vi "Define PDE Boundary Condition.vi"   [LabVIEW 2017, in "NI_PDE.lvlib"]
doc: "Defines the boundary condition of partial differential equations. You must manually select the polymorphic instance to use."
uses:
  <vilib>/gmath/NI_PDE.lvlib
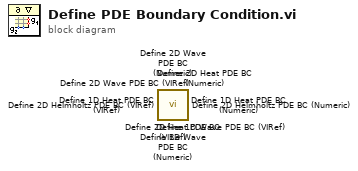
[diagram p0: block diagram]
diagram:
  n1 = call <vilib>:"Define 2D Heat PDE BC (VIRef).vi"() -> ()  [unwired: 14 in, 2 out]
  n2 = call <vilib>:"Define 2D Heat PDE BC (Numeric).vi"() -> ()  [unwired: 14 in, 2 out]
  n3 = call <vilib>:"Define 1D Heat PDE BC (VIRef).vi"() -> ()  [unwired: 14 in, 2 out]
  n4 = call <vilib>:"Define 1D Heat PDE BC (Numeric).vi"() -> ()  [unwired: 14 in, 2 out]
  n5 = call <vilib>:"Define 2D Wave PDE BC (VIRef).vi"() -> ()  [unwired: 14 in, 2 out]
  n6 = call <vilib>:"Define 2D Wave PDE BC (Numeric).vi"() -> ()  [unwired: 14 in, 2 out]
  n7 = call <vilib>:"Define 1D Wave PDE BC (VIRef).vi"() -> ()  [unwired: 14 in, 2 out]
  n8 = call <vilib>:"Define 1D Wave PDE BC (Numeric).vi"() -> ()  [unwired: 14 in, 2 out]
  n9 = call <vilib>:"Define 2D Helmholtz PDE BC (VIRef).vi"() -> ()  [unwired: 14 in, 2 out]
  n10 = call <vilib>:"Define 2D Helmholtz PDE BC (Numeric).vi"() -> ()  [unwired: 14 in, 2 out]
